vi "Wait End.vi"(8 "error in (no error)":errorcluster caption="entrée d'erreur (pas d'erreur)", 11 "Process (Default) en entrée":refnum<class "Process (Default).lvclass">) -> (0 "error out":errorcluster caption="sortie d'erreur", 3 "Process (Default) en sortie":refnum<class "Process (Default).lvclass">)   [LabVIEW 2020, in "Library Instrument & Equipement.lvlib" / "Process (Default).lvclass"]
uses:
  Process (Default).lvclass
  Process (Default).lvclass/Process (Default).ctl
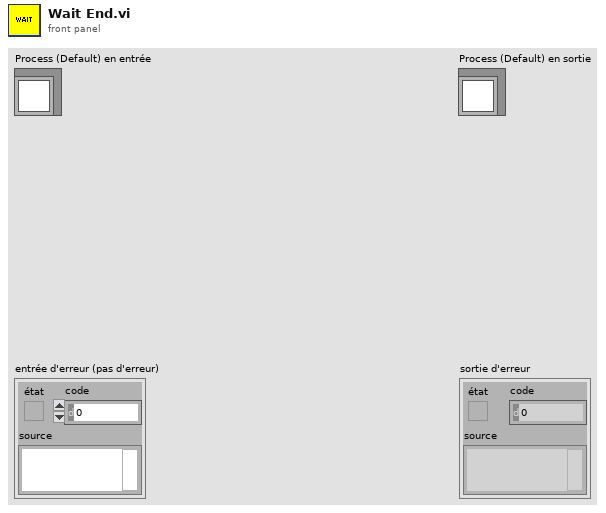
[diagram p1: front panel]
types:
  T1 = cluster{"Standard Output":string, "Process_is_Finish":bool}
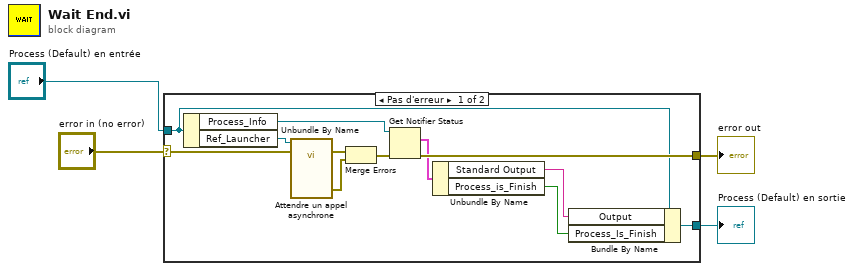
[diagram p0: block diagram]
diagram:
  n1 = case shown="Pas d'erreur" "error in (no error)" {
    selector: "error in (no error)" -> [w13 w18]
    tunnel: [w11 w18] -> w3
    tunnel: [w8 w17] -> w1
    tunnel: "Process (Default) en entrée" -> [w9 w17]
    frame No Error {
      n2 = Unbundle By Name(w9) -> ("Process_Info"=w10:refnum<notifier>, "Ref_Launcher"=w16:refnum<vi>)
      n3 = call-by-ref "Attendre un appel asynchrone"(reference=w16, error in=w13) -> (error out=w15:errorcluster, 0:"error out"=w14:errorcluster)  [unwired: 11 in, 1 out]
      n4 = Merge Errors(w15, w14) -> (w12:errorcluster)
      n5 = Get Notifier Status(notifier=w10, error in (no error)=w12) -> (current notification=w7:T1, error out=w11:errorcluster)  [unwired: 3 out]
      n6 = Unbundle By Name(w7) -> ("Standard Output"=w6:string, "Process_is_Finish"=w5:bool)
      n7 = Bundle By Name(cluster=w9, "Output"=w6, "Process_Is_Finish"=w5) -> (w8:refnum<class "Process (Default).lvclass">)
    }
    frame Error {
    }
  }
  "error out" <- w3
  "Process (Default) en sortie" <- w1
